vi "Add Controls in Result.vi"(0 "vi reference":refnum<vi>, 5 "result cluster":refnum<vi>, 7 "new code module":path, 11 "error in":errorcluster) -> (15 "error out":errorcluster)   [LabVIEW 2021, in "Converter.lvlib"]
uses:
  Converter.lvlib
  Converter Reusables/Converter Reusables.lvlib
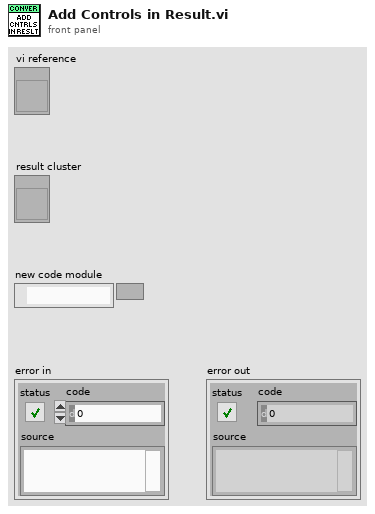
[diagram p1: front panel]
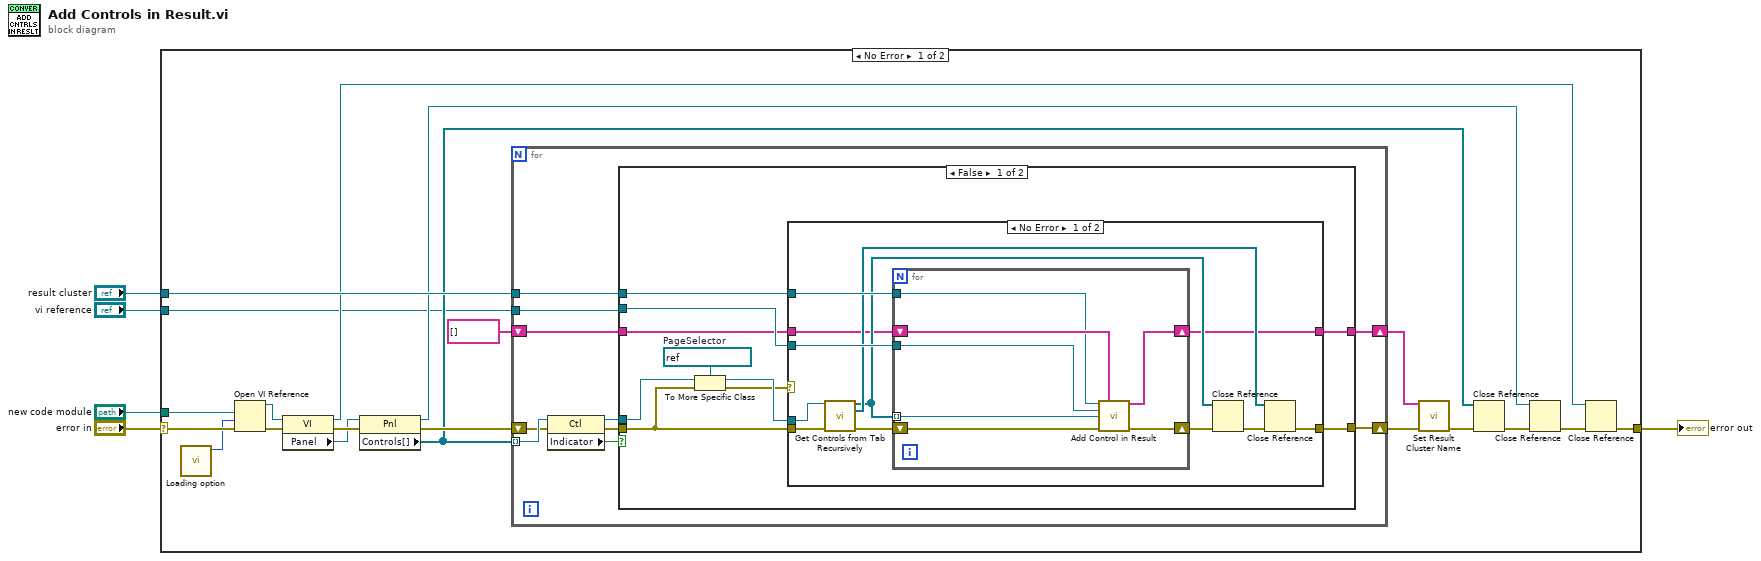
[diagram p0: block diagram]
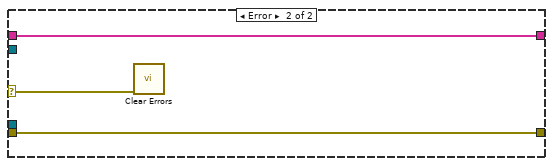
[diagram p2: hidden frame]
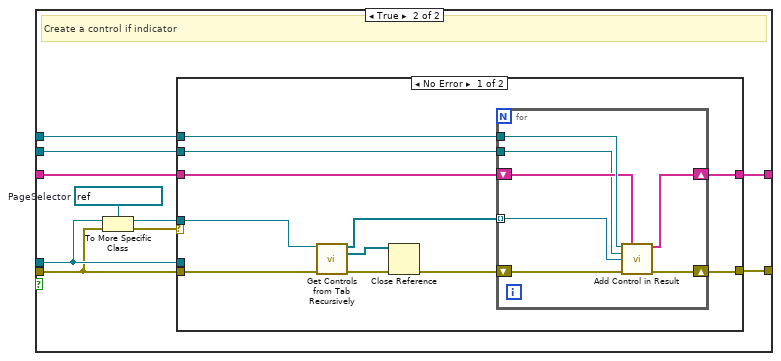
[diagram p3: hidden frame]
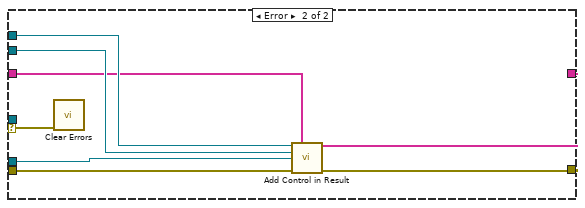
[diagram p4: hidden frame]
diagram:
  n1 = case shown="No Error" "error in" {
    selector: "error in" -> [w25 w104]
    tunnel: "new code module" -> [w24 _]
    tunnel: "result cluster" -> [w23 _]
    tunnel: [w15 w104] -> w2
    tunnel: "vi reference" -> [w11 _]
    frame No Error {
      n2 = call "Loading option.vi"() -> ("options"=w6:i32)  [unwired: 11 in]
      n3 = Open VI Reference(vi path=w24, options=w6, error in (no error)=w25) -> (vi reference=w16:refnum<vi>, error out=w20:errorcluster)  [unwired: 3 in]
      n4 = property class="VI"(reference=w16, error in=w20) -> (reference out=w13:refnum<vi>, error out=w21:errorcluster, "Panel"=w18:refnum<vi>)
      n5 = property class="Pnl"(reference=w18, error in=w21) -> (reference out=w12:refnum<vi>, error out=w22:errorcluster, "Controls[]"=w19:refnum<vi>[])
      n6 = for {
        tunnel: w19 -> [w33] mode=indexing
        shift-right: [w34] -> w7
        shift-left: w22 -> [w31]
        tunnel: w23 -> [w35]
        tunnel: w11 -> [w28]
        shift-right: [w27] -> w9
        shift-left: string[] [] ("Output Clusters") -> [w26]
        n7 = property class="Ctl"(reference=w33, error in=w31) -> (reference out=w29:refnum<vi>, error out=w30:errorcluster, "Indicator"=w32:bool)
        n8 = case shown="False" w32 {
          tunnel: w35 -> [w38 w77]
          tunnel: w30 -> [w40 w73]
          tunnel: w29 -> [w45 w74]
          tunnel: [w42 w76] -> w34
          tunnel: w28 -> [w41 w75]
          tunnel: [w36 w69] -> w27
          tunnel: w26 -> [w37 w68]
          frame False {
            w44 = refnum<vi> refnum  # PageSelector
            n9 = To More Specific Class(target class=w44, reference=w45, error in=w40) -> (specific class reference=w43:refnum<vi>, error out=w39:errorcluster)
            n10 = case shown="No Error" w39 {
              selector: w39 -> [_ w67]
              tunnel: w43 -> [w57 _]
              tunnel: [w53 w66] -> w42
              tunnel: w41 -> [w52 _]
              tunnel: w40 -> [w51 w66]
              tunnel: w38 -> [w50 _]
              tunnel: w37 -> [w47 w65]
              tunnel: [w46 w65] -> w36
              frame No Error {
                n11 = call "Get Controls from Tab Recursively.vi"("page sel refnum"=w57, "error in"=w51) -> ("indicators in tab"=w48:refnum<vi>[], "controls in tab"=w49:refnum<vi>[], "error out"=w56:errorcluster)  [unwired: 11 in]
                n12 = for {
                  shift-right: [w59] -> w55
                  shift-left: w56 -> [w58]
                  tunnel: w48 -> [w60] mode=indexing
                  tunnel: w52 -> [w61]
                  tunnel: w50 -> [w62]
                  shift-right: [w63] -> w46
                  shift-left: w47 -> [w64]
                  n13 = call "Add Control in Result.vi"("result cluster"=w62, "output clusters in"=w64, "vi reference"=w61, "ctl refnum"=w60, "error in"=w58) -> ("output clusters out"=w63:string[], "error out"=w59:errorcluster)  [unwired: 9 in]
                }
                n14 = Close Reference(reference=w48, error in (no error)=w55) -> (error out=w54:errorcluster)
                n15 = Close Reference(reference=w49, error in (no error)=w54) -> (error out=w53:errorcluster)
              }
              frame Error {
                n16 = call <vilib>:"Clear Errors.vi"("error in (no error)"=w67) -> ()  [unwired: 5 in, 2 out]
              }
            }
          }
          frame True {
            w72 = refnum<vi> refnum  # PageSelector
            # "Create a control if indicator"
            n17 = To More Specific Class(target class=w72, reference=w74, error in=w73) -> (specific class reference=w70:refnum<vi>, error out=w71:errorcluster)
            n18 = case shown="No Error" w71 {
              selector: w71 -> [_ w100]
              tunnel: w77 -> [w82 w103]
              tunnel: [w80 w102] -> w76
              tunnel: w75 -> [w81 w101]
              tunnel: w74 -> [_ w99]
              tunnel: w73 -> [w87 w96]
              tunnel: w70 -> [w88 _]
              tunnel: [w78 w98] -> w69
              tunnel: w68 -> [w79 w97]
              frame No Error {
                n19 = call "Get Controls from Tab Recursively.vi"("page sel refnum"=w88, "error in"=w87) -> ("indicators in tab"=w84:refnum<vi>[], "controls in tab"=w86:refnum<vi>[], "error out"=w85:errorcluster)  [unwired: 11 in]
                n20 = Close Reference(reference=w86, error in (no error)=w85) -> (error out=w83:errorcluster)
                n21 = for {
                  tunnel: w84 -> [w93] mode=indexing
                  tunnel: w82 -> [w94]
                  shift-right: [w92] -> w80
                  shift-left: w83 -> [w95]
                  tunnel: w81 -> [w89]
                  shift-right: [w90] -> w78
                  shift-left: w79 -> [w91]
                  n22 = call "Add Control in Result.vi"("result cluster"=w94, "output clusters in"=w91, "vi reference"=w89, "ctl refnum"=w93, "error in"=w95) -> ("output clusters out"=w90:string[], "error out"=w92:errorcluster)  [unwired: 9 in]
                }
              }
              frame Error {
                n23 = call <vilib>:"Clear Errors.vi"("error in (no error)"=w100) -> ()  [unwired: 5 in, 2 out]
                n24 = call "Add Control in Result.vi"("result cluster"=w103, "output clusters in"=w97, "vi reference"=w101, "ctl refnum"=w99, "error in"=w96) -> ("output clusters out"=w98:string[], "error out"=w102:errorcluster)  [unwired: 9 in]
              }
            }
          }
        }
      }
      n25 = call "Set Result Cluster Name.vi"("controls name"=w9, "error in"=w7) -> ("error out"=w8:errorcluster)  [unwired: 13 in]
      n26 = Close Reference(reference=w19, error in (no error)=w8) -> (error out=w17:errorcluster)
      n27 = Close Reference(reference=w12, error in (no error)=w17) -> (error out=w14:errorcluster)
      n28 = Close Reference(reference=w13, error in (no error)=w14) -> (error out=w15:errorcluster)
    }
    frame Error {
    }
  }
  "error out" <- w2
